vi "Read RT FIFO.vi"(7 "FIFO Options":T1, 8 "error in (no error)":errorcluster, 9 "timeout in ms (0)":i32, 11 "RT FIFO in":T2) -> (0 "error out":errorcluster, 1 "empty?":bool, 2 "element out":T3, 3 "RT FIFO out":T2, 4 "# elements":u32)   [LabVIEW 2017, in "DSF Core.lvlib" / "Interface.lvclass"]
uses:
  Interface.lvclass
  RT FIFO Data.ctl
  RT FIFO Parameters.ctl
  RT FIFO Ref.ctl
  Typedefs/FIFO Flags.ctl
  DSF Core.lvlib
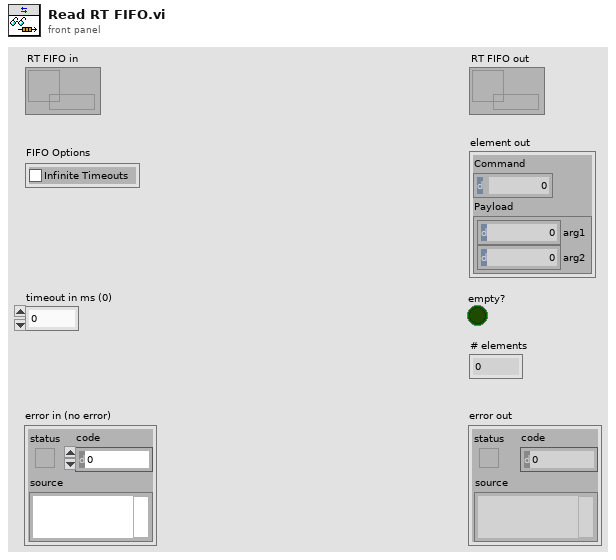
[diagram p1: front panel]
types:
  T1 = typedef "DSF Core.lvlib/FIFO Flags.ctl" = cluster{"Infinite Timeouts":bool}
  T2 = typedef "DSF Core.lvlib/Interface.lvclass/RT FIFO Ref.ctl" = refnum<k33>
  T3 = typedef "DSF Core.lvlib/Interface.lvclass/RT FIFO Data.ctl" = cluster{"Command":u8, "Payload":T4}
  T4 = typedef "DSF Core.lvlib/Interface.lvclass/RT FIFO Parameters.ctl" = cluster{"arg1":u64, "arg2":u64}
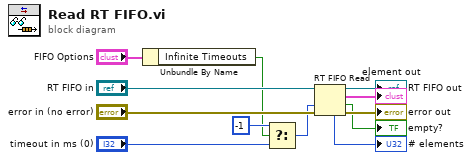
[diagram p0: block diagram]
diagram:
  n1 = Unbundle By Name("FIFO Options") -> ("Infinite Timeouts"=w1:bool)
  n2 = Select(t=-1, s=w1, f="timeout in ms (0)") -> (s? t:f=w3:i32)
  n3 = RT FIFO Read(0:"RT FIFO in", 2:w3, 3:"error in (no error)") -> (7:→"# elements":u32, 8:→"RT FIFO out":T2, 9:→"element out":T3, 10:→"empty?":bool, 11:→"error out":errorcluster)  [unwired: 1 in]
